vi "Single SSC DCPower Configure Single Point Force DC Current Asymmetric Limits.vi"(0 "DCPower SSC in":T1, 1 "Current Level Range (A)":dbl format="%#_6p", 2 "Voltage Limit Range (V)":dbl format="%#_6p", 5 "Current Level (A)":dbl format="%#_6p", 7 "Voltage Limit High (V)":dbl format="%#_6p", 9 "Voltage Limit Low (V)":dbl format="%#_6p", 11 "error in":errorcluster) -> (4 "DCPower SSC out":T1, 15 "error out":errorcluster)   [LabVIEW 2020]
doc: "This VI configures the sessions to force a single point DC current level with asymmetric voltage limits."
uses:
  SSC DCPower.ctl
  <instrlib>/niDCPower/nidcpower.llb/niDCPower Source Mode.ctl
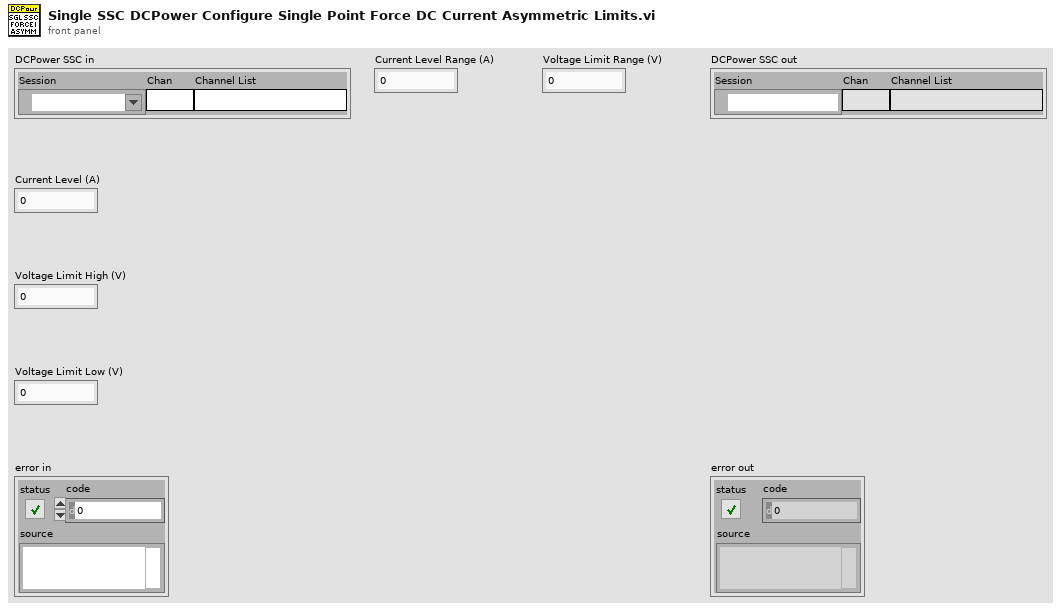
[diagram p1: front panel]
types:
  T1 = typedef "SSC DCPower.ctl" = cluster{"Session":refnum<k15>, "Chan":string, "Channel List":string}
  T2 = typedef "niDCPower Source Mode.ctl" = i32
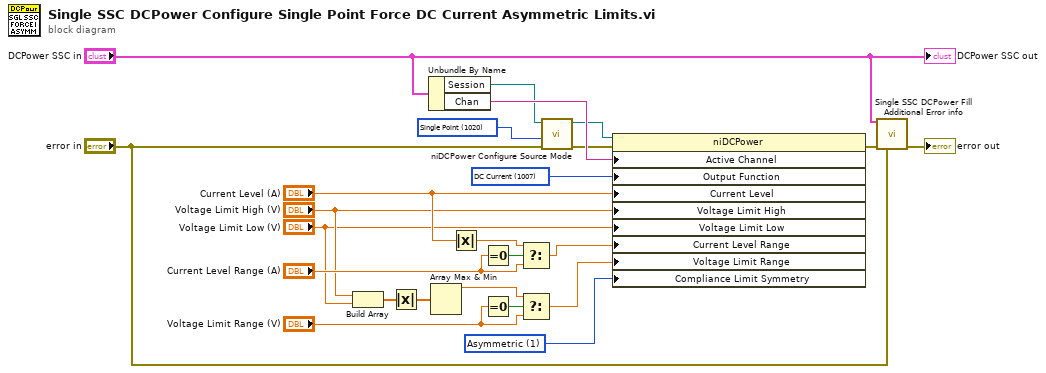
[diagram p0: block diagram]
diagram:
  w6 = 1 items=["Symmetric", "Asymmetric"] ("Source:Advanced:Compliance Limit Symmetry")
  w10 = T2 1020 items=["Single Point"=1020, "Sequence"=1021] ("source mode")
  w14 = 1007 items=["DC Voltage"=1006, "DC Current"=1007, "Pulse Voltage"=1049, "Pulse Current"=1050] ("Source:Output Function")
  n1 = Build Array("Voltage Limit High (V)", "Voltage Limit Low (V)") -> (w3:dbl[])
  n2 = Absolute Value(x=w3) -> (abs(x)=w1:dbl[])
  n3 = Unbundle By Name("DCPower SSC in") -> ("Session"=w12:refnum<k15>, "Chan"=w15:string)
  n4 = Array Max & Min(array=w1) -> (max value=w2:dbl)  [unwired: 3 out]
  n5 = Absolute Value(x="Current Level (A)") -> (abs(x)=w24:dbl)
  n6 = Equal To 0?(x="Current Level Range (A)") -> (x = 0?=w23:bool)
  n7 = Equal To 0?(x="Voltage Limit Range (V)") -> (x = 0?=w22:bool)
  n8 = Select(t=w24, s=w23, f="Current Level Range (A)") -> (s? t:f=w21:dbl)
  n9 = Select(t=w2, s=w22, f="Voltage Limit Range (V)") -> (s? t:f=w20:dbl)
  n10 = call <instrlib>:"niDCPower Configure Source Mode.vi"("error in (no error)"="error in", "source mode"=w10, "instrument handle"=w12) -> ("error out"=w13:errorcluster, "instrument handle out"=w11:refnum<k15>)  [unwired: 7 in]
  n11 = property class="niDCPower"(reference=w11, error in=w13, "Active Channel"=w15, "Output Function"=w14, "Current Level"="Current Level (A)", "Voltage Limit High"="Voltage Limit High (V)", "Voltage Limit Low"="Voltage Limit Low (V)", "Current Level Range"=w21, "Voltage Limit Range"=w20, "Compliance Limit Symmetry"=w6) -> (error out=w19:errorcluster)  [unwired: 1 out]
  n12 = call "Single SSC DCPower Fill Additional Error info.vi"("DCPower SSC in"="DCPower SSC in", "error in"=w19, "previous error in"="error in") -> ("error out"=→"error out":errorcluster)  [unwired: 12 in]
  "DCPower SSC out" <- "DCPower SSC in"
